vi "LEFT.vi"() -> (3 "LEFT":cluster{"x":i16, "y":i16})   [LabVIEW 2025, in "AOC.lvlib"]
uses:
  AOC/AOC.lvlib
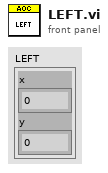
[diagram p1: front panel]
types:
  T1 = cluster{"unsigned 8bit integer":i16, "unsigned 8bit integer":i16}
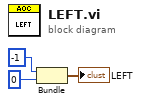
[diagram p0: block diagram]
diagram:
  n1 = Bundle("unsigned 8bit integer"=i16 -1, "unsigned 8bit integer"=i16 0) -> (→"LEFT":T1)  [unwired: 1 in]
